vi "Enqueue_Elements.vi"(6 "Prioritize?":bool, 8 "error in (no error)":errorcluster, 9 "Data":variant, 10 "State":T1, 11 "Queue in":refnum<queue>) -> (0 "error out":errorcluster)   [LabVIEW 2023]
doc: "This VI enqueues the elements if prioritize is true it puts the elemtns on opposite end"
uses:
  Controls/State.ctl
  Controls/Queued_Data.ctl
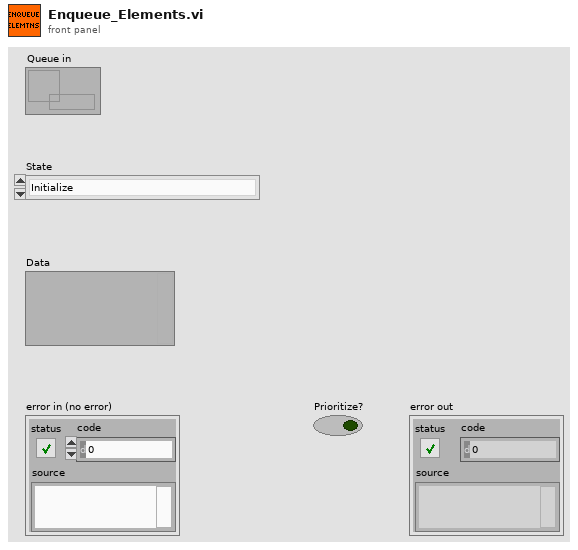
[diagram p1: front panel]
types:
  T1 = typedef "State.ctl" = enum16{"Initialize", "Save Wash Options", "Start Process", "Car Position", "Order Steps to follow", "Under Body Wash", "Bug Remover", "Pre-Soak", "Stop Application"}
  T2 = typedef "Queued_Data.ctl" = cluster{"State":T1, "Data":variant}
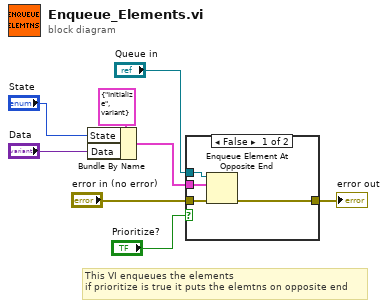
[diagram p0: block diagram]
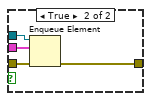
[diagram p2: hidden frame]
diagram:
  # "This VI enqueues the elements\nif prioritize is true it puts the elemtns on opposite end"
  n1 = Bundle By Name(cluster=T2 {"State"=enum."Initialize", "Data"=variant}, "State"="State", "Data"="Data") -> (w7:T2)
  n2 = case shown="False" "Prioritize?" {
    tunnel: w7 -> [w9 w16]
    tunnel: [w11 w15] -> w6
    tunnel: "error in (no error)" -> [w12 w14]
    tunnel: "Queue in" -> [w10 w13]
    frame False {
      n3 = Enqueue Element At Opposite End(queue=w10, element=w9, error in (no error)=w12) -> (error out=w11:errorcluster)  [unwired: 1 in, 2 out]
    }
    frame True {
      n4 = Enqueue Element(queue=w13, element=w16, error in (no error)=w14) -> (error out=w15:errorcluster)  [unwired: 1 in, 2 out]
    }
  }
  "error out" <- w6
